vi "Play Sound.vi"(8 "error in (no error)":errorcluster, 9 "Enable Sound":bool, 10 "Volume":dbl(knob) scale=0.0..2000.0, 11 "Electrophysiology in":refnum<class "Behavior.lvclass">) -> (0 "error out":errorcluster, 3 "Electrophysiology out":refnum<class "Behavior.lvclass">)   [LabVIEW 2010]
uses:
  <vilib>/sound2/lvsound2.llb/Sound Output Write (DBL).vi
  Behavior.lvclass
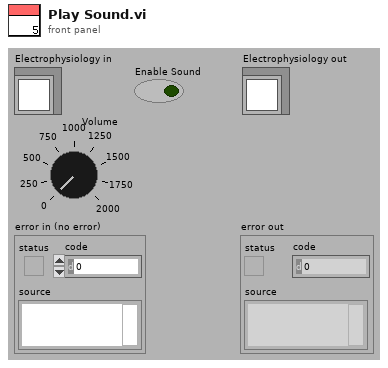
[diagram p1: front panel]
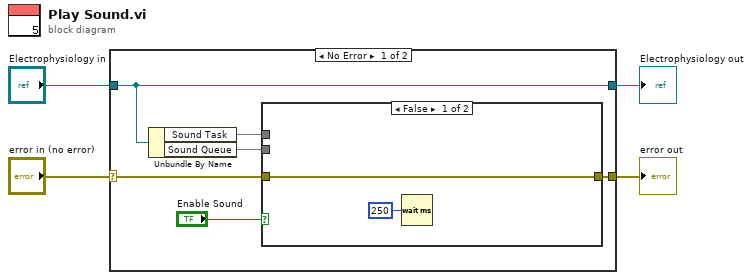
[diagram p0: block diagram]
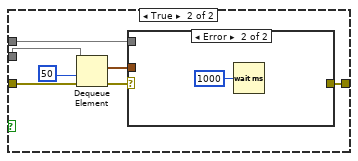
[diagram p2: hidden frame]
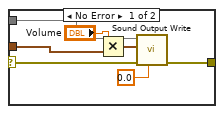
[diagram p3: hidden frame]
diagram:
  n1 = case shown="No Error" "error in (no error)" {
    selector: "error in (no error)" -> [w8 w29]
    tunnel: [w7 w29] -> w3
    tunnel: [w10 w28] -> w1
    tunnel: "Electrophysiology in" -> [w10 w28]
    frame No Error {
      n2 = Unbundle By Name(w10) -> ("Sound Task"=w9, "Sound Queue"=w6)
      n3 = case shown="False" "Enable Sound" {
        tunnel: w9 -> [_ w19]
        tunnel: w8 -> [w12 w18]
        tunnel: [w12 w17] -> w7
        tunnel: w6 -> [_ w15]
        frame False {
          n4 = Wait (ms)(milliseconds to wait=u32 250) -> ()  [unwired: 1 out]
        }
        frame True {
          n5 = Dequeue Element(queue=w15, timeout in ms (-1)=u32 50 ("milliseconds to wait"), error in (no error)=w18) -> (element=w16:waveform(dbl)[], error out=w14:errorcluster)  [unwired: 2 out]
          n6 = case shown="Error" w14 {
            selector: w14 -> [w20 _]
            tunnel: w19 -> [w24 _]
            tunnel: [w23 _] -> w17
            tunnel: w16 -> [w22 _]
            frame No Error {
              n7 = Multiply(x="Volume", y=w22) -> (x*y=w26:waveform(dbl)[])
              n8 = call-poly <vilib>:"Sound Output Write.vi"("timeout (sec)"=0.0, "error in (no error)"=w20, "data"=w26, "task ID"=w24) -> ("error out"=w23:errorcluster)  [unwired: 6 in, 1 out]
            }
            frame Error {
              n9 = Wait (ms)(milliseconds to wait=u32 1000) -> ()  [unwired: 1 out]
            }
          }
        }
      }
    }
    frame Error {
    }
  }
  "error out" <- w3
  "Electrophysiology out" <- w1
